vi "Draw Project Results Table.vi"(8 "error in":errorcluster, 9 "Project Results":string[][](array[string]), 11 "Project Results Ref":refnum<vi>) -> (0 "error out":errorcluster)   [LabVIEW 2019, in "Panther Dashboard.lvlib"]
uses:
  Panther Dashboard.lvlib
  <vilib>/Utility/miscctls.llb/LVRowAndColumnTypeDef.ctl
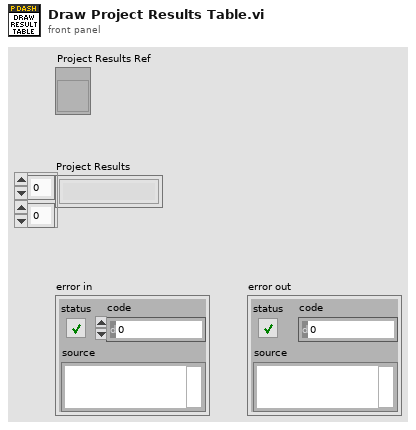
[diagram p1: front panel]
types:
  T1 = typedef "LVRowAndColumnTypeDef.ctl" = cluster{"Row":i32, "Column":i32}
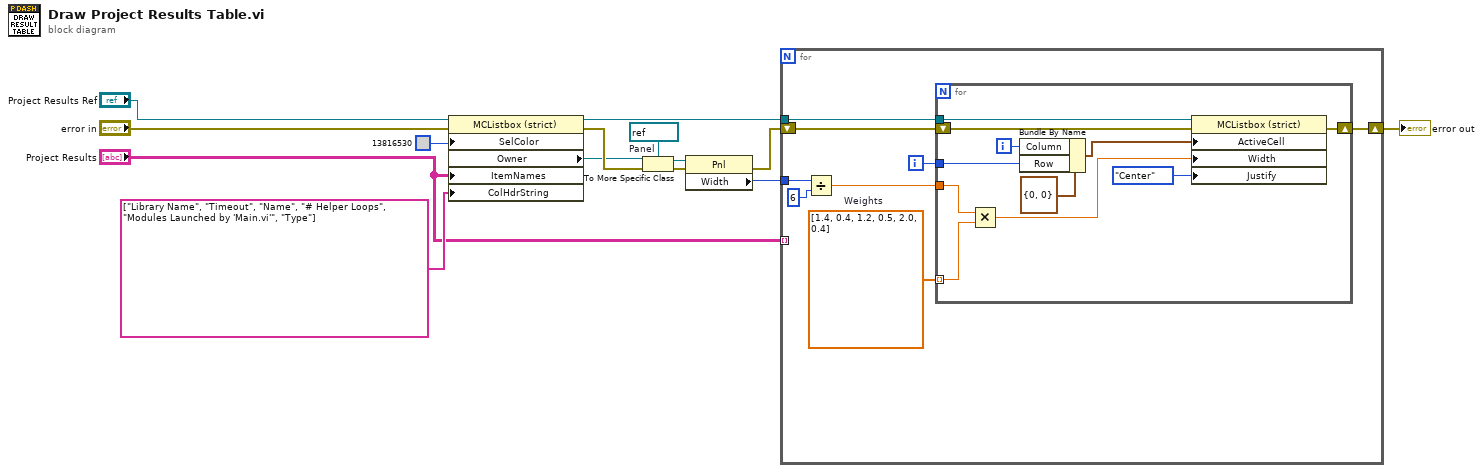
[diagram p0: block diagram]
diagram:
  w7 = refnum<vi> refnum  # Panel
  n1 = property on="Property Node" class="MCListbox (strict)"(reference="Project Results Ref", error in="error in", "SelColor"=u32 13816530, "ItemNames"="Project Results", "ColHdrString"=string[] ["Library Name", "Timeout", "Name", "# Helper Loops", "Modules Launched by 'Main.vi'", "Type"] ("Column Header Strings[]")) -> (reference out=w6:refnum<vi>, error out=w12:errorcluster, "Owner"=w3:refnum<vi>)
  n2 = To More Specific Class(target class=w7, reference=w3, error in=w12) -> (specific class reference=w8:refnum<vi>, error out=w13:errorcluster)
  n3 = property class="Pnl"(reference=w8, error in=w13) -> (error out=w14:errorcluster, "Width"=w9:u32)  [unwired: 1 out]
  n4 = for {
    tunnel: w9 -> [w19]
    tunnel: w6 -> [w18]
    shift-right: [w21] -> w10
    shift-left: w14 -> [w22]
    tunnel: "Project Results" -> [_] mode=indexing
    i -> [w17]
    w16 = dbl[] [1.4, 0.4, 1.2, 0.5, 2.0, 0.4]  # Weights
    n5 = Divide(x=w19, y=u32 6) -> (x/y=w20:dbl)
    n6 = for {
      tunnel: w20 -> [w29]
      tunnel: w16 -> [w27] mode=indexing
      tunnel: w18 -> [w26]
      shift-right: [w32] -> w21
      shift-left: w22 -> [w33]
      tunnel: w17 -> [w25]
      i -> [w30]
      n7 = Multiply(x=w29, y=w27) -> (x*y=w28:dbl)
      n8 = Bundle By Name(cluster=T1 {"Row"=0, "Column"=0} ("Active Cell:Active Cell"), "Column"=w30, "Row"=w25) -> (w31:T1)
      n9 = property class="MCListbox (strict)"(reference=w26, error in=w33, "ActiveCell"=w31, "Width"=w28, "Justify"=enum16{"Left", "Center", "Right"}."Center" ("Active Cell:Cell Justification")) -> (error out=w32:errorcluster)  [unwired: 1 out]
    }
  }
  "error out" <- w10
